vi "GasLines Control.vi"(9 "Numeric 2":u16, 10 "Numeric":u16, 11 "Array":refnum<vi>[][](array[refnum])) -> ()   [LabVIEW 2020]
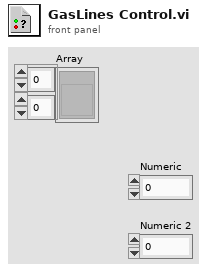
[diagram p1: front panel]
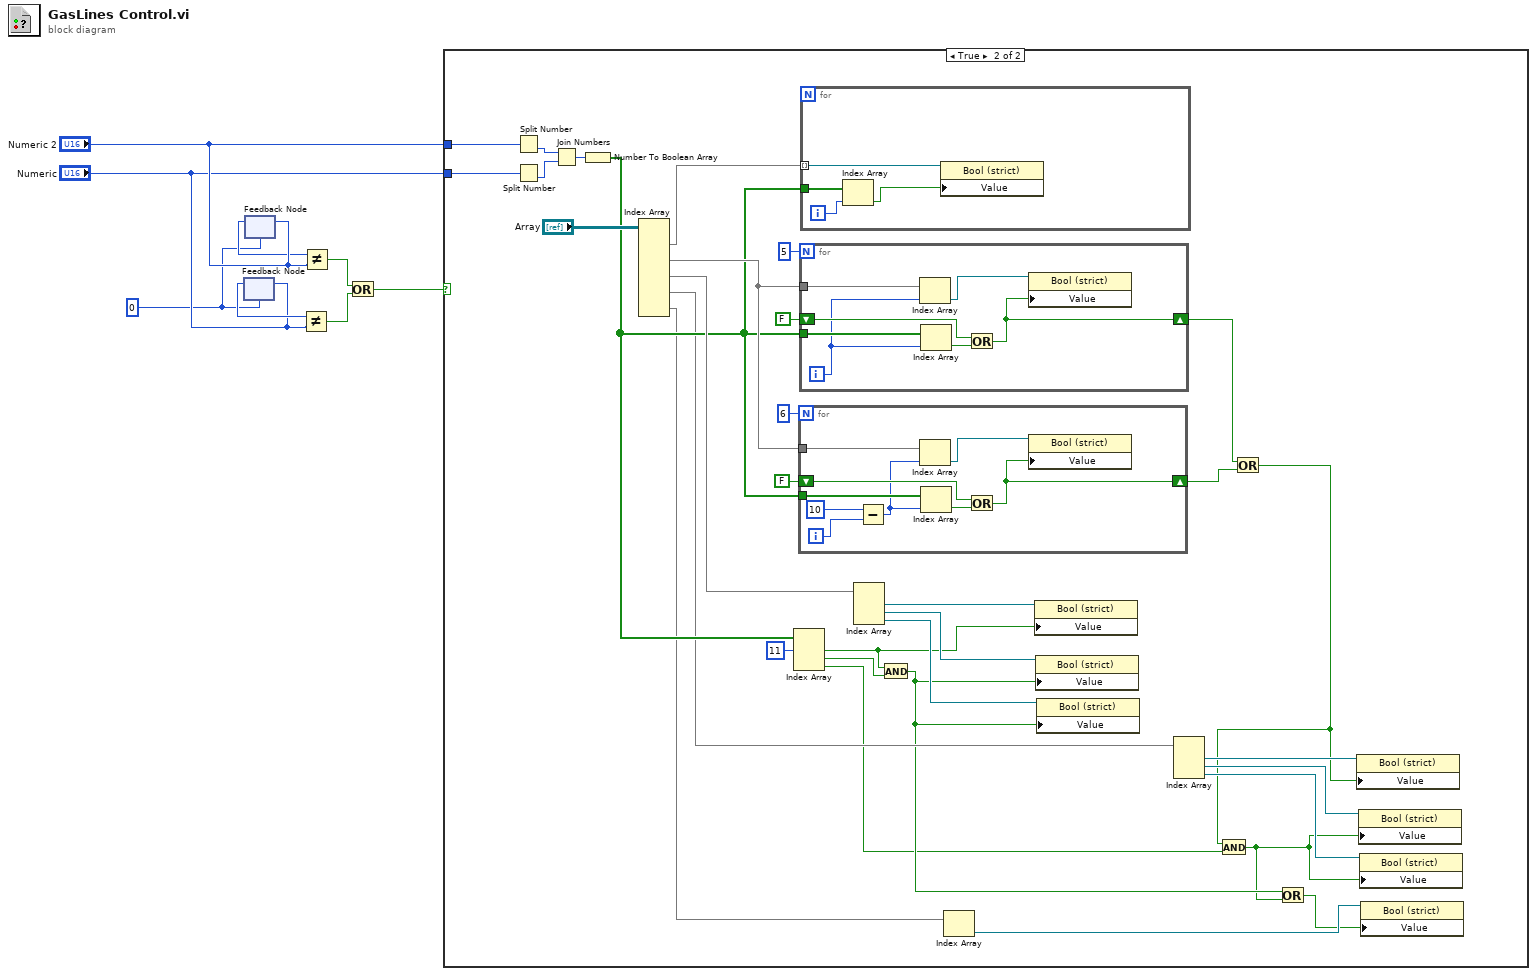
[diagram p0: block diagram]
diagram:
  w1 = u16 0 ("Numeric")
  n1 = feedback #1(w1) -> (w6:u16)
  n2 = feedback-in #1("Numeric") -> ()
  n3 = feedback-in #2("Numeric 2") -> ()
  n4 = feedback #2(w1) -> (w7:u16)
  n5 = Not Equal?(x=w6, y="Numeric") -> (x != y?=w3:bool)
  n6 = Not Equal?(x=w7, y="Numeric 2") -> (x != y?=w4:bool)
  n7 = Or(x=w4, y=w3) -> (x .or. y?=w2:bool)
  n8 = case shown="True" w2 {
    tunnel: "Numeric 2" -> [_ w37]
    tunnel: "Numeric" -> [_ w36]
    frame False {
    }
    frame True {
      n9 = Split Number(x=w37) -> (lo(x)=w39:u8)  [unwired: 1 out]
      n10 = Split Number(x=w36) -> (lo(x)=w38:u8)  [unwired: 1 out]
      n11 = Join Numbers(hi=w39, lo=w38) -> ((hi.lo)=w40:u16)
      n12 = Number To Boolean Array(number=w40) -> (Boolean array=w28:bool[])
      n13 = Index Array(array="Array") -> (element #1=w30:refnum<vi>[], element #2=w31:refnum<vi>[], element #3=w29:refnum<vi>[], element #4=w20:refnum<vi>[], element #5=w19:refnum<vi>[])  [unwired: 10 in]
      n14 = Index Array(array=w28, index #1=11 ("index")) -> (element #1=w16:bool, element #2=w15:bool, element #3=w13:bool)  [unwired: 2 in]
      n15 = for {
        N: 6 -> [_]
        tunnel: w28 -> [w54]
        shift-right: [w49] -> w11
        shift-left: FALSE -> [w52]
        tunnel: w31 -> [w51]
        i -> [w48]
        n16 = Subtract(x=10, y=w48) -> (x-y=w46:i32)
        n17 = Index Array(array=w51, index=w46) -> (element=w50:refnum<vi>)
        n18 = Index Array(array=w54, index=w46) -> (element=w53:bool)
        n19 = Or(x=w52, y=w53) -> (x .or. y?=w49:bool)
        n20 = property class="Bool (strict)"(reference=w50, "Value"=w49) -> ()  [unwired: 1 in, 2 out]
      }
      n21 = for {
        N: 5 -> [_]
        tunnel: w28 -> [w61]
        shift-right: [w55] -> w10
        shift-left: FALSE -> [w59]
        tunnel: w31 -> [w58]
        i -> [w57]
        n22 = Index Array(array=w58, index=w57) -> (element=w56:refnum<vi>)
        n23 = Index Array(array=w61, index=w57) -> (element=w60:bool)
        n24 = Or(x=w59, y=w60) -> (x .or. y?=w55:bool)
        n25 = property class="Bool (strict)"(reference=w56, "Value"=w55) -> ()  [unwired: 1 in, 2 out]
      }
      n26 = for {
        tunnel: w30 -> [w45] mode=indexing
        tunnel: w28 -> [w43]
        i -> [w44]
        n27 = Index Array(array=w43, index=w44) -> (element=w42:bool)
        n28 = property class="Bool (strict)"(reference=w45, "Value"=w42) -> ()  [unwired: 1 in, 2 out]
      }
      n29 = Index Array(array=w29) -> (element #1=w26:refnum<vi>, element #2=w25:refnum<vi>, element #3=w24:refnum<vi>)  [unwired: 3 in]
      n30 = And(x=w16, y=w15) -> (x .and. y?=w14:bool)
      n31 = Index Array(array=w19) -> (element=w18:refnum<vi>)  [unwired: 1 in]
      n32 = property class="Bool (strict)"(reference=w26, "Value"=w16) -> ()  [unwired: 1 in, 2 out]
      n33 = property class="Bool (strict)"(reference=w25, "Value"=w14) -> ()  [unwired: 1 in, 2 out]
      n34 = property class="Bool (strict)"(reference=w24, "Value"=w14) -> ()  [unwired: 1 in, 2 out]
      n35 = Index Array(array=w20) -> (element #1=w21:refnum<vi>, element #2=w22:refnum<vi>, element #3=w23:refnum<vi>)  [unwired: 3 in]
      n36 = Or(x=w10, y=w11) -> (x .or. y?=w9:bool)
      n37 = And(x=w9, y=w13) -> (x .and. y?=w12:bool)
      n38 = Or(x=w14, y=w12) -> (x .or. y?=w17:bool)
      n39 = property class="Bool (strict)"(reference=w21, "Value"=w9) -> ()  [unwired: 1 in, 2 out]
      n40 = property class="Bool (strict)"(reference=w22, "Value"=w12) -> ()  [unwired: 1 in, 2 out]
      n41 = property class="Bool (strict)"(reference=w23, "Value"=w12) -> ()  [unwired: 1 in, 2 out]
      n42 = property class="Bool (strict)"(reference=w18, "Value"=w17) -> ()  [unwired: 1 in, 2 out]
    }
  }
